vi "Power Qualtiy - 7 (Sub Vi).vi"(8 "Dynamic Data 6":dynamicdata(waveform)) -> (10 "Dynamic Data 2":dynamicdata(waveform), 12 "Dynamic Data":dynamicdata(waveform), 14 "Dynamic Data 4":dynamicdata(waveform), 15 "FFT - (RMS)":dynamicdata(waveform), 16 "Current":dbl(knob) scale=0.0..10.0, 17 "RMS":dynamicdata(waveform), 18 "Current Harmonics":dynamicdata(graph), 19 "IHD 7":dbl, 20 "Dynamic Data 3":dynamicdata(waveform), 21 "THD":dbl, 22 "Dynamic Data 5":dynamicdata(waveform), 23 "IHD 1":dbl, 24 "THD 2":dynamicdata(waveform), 25 "IHD 3":dbl, 26 "IHD 5":dbl)   [LabVIEW 2015]
uses:
  <vilib>/express/express analysis/Spectral/Block/exnSpectralBlock spectral measurements RMS poly.vi
  <vilib>/express/express analysis/Spectral/Block/exnSpectralBlock spectral measurements RMS DDT.vi
  <vilib>/express/express analysis/Spectral/XNode/ExpressSpectralMeasurementsBlockNode.xnode
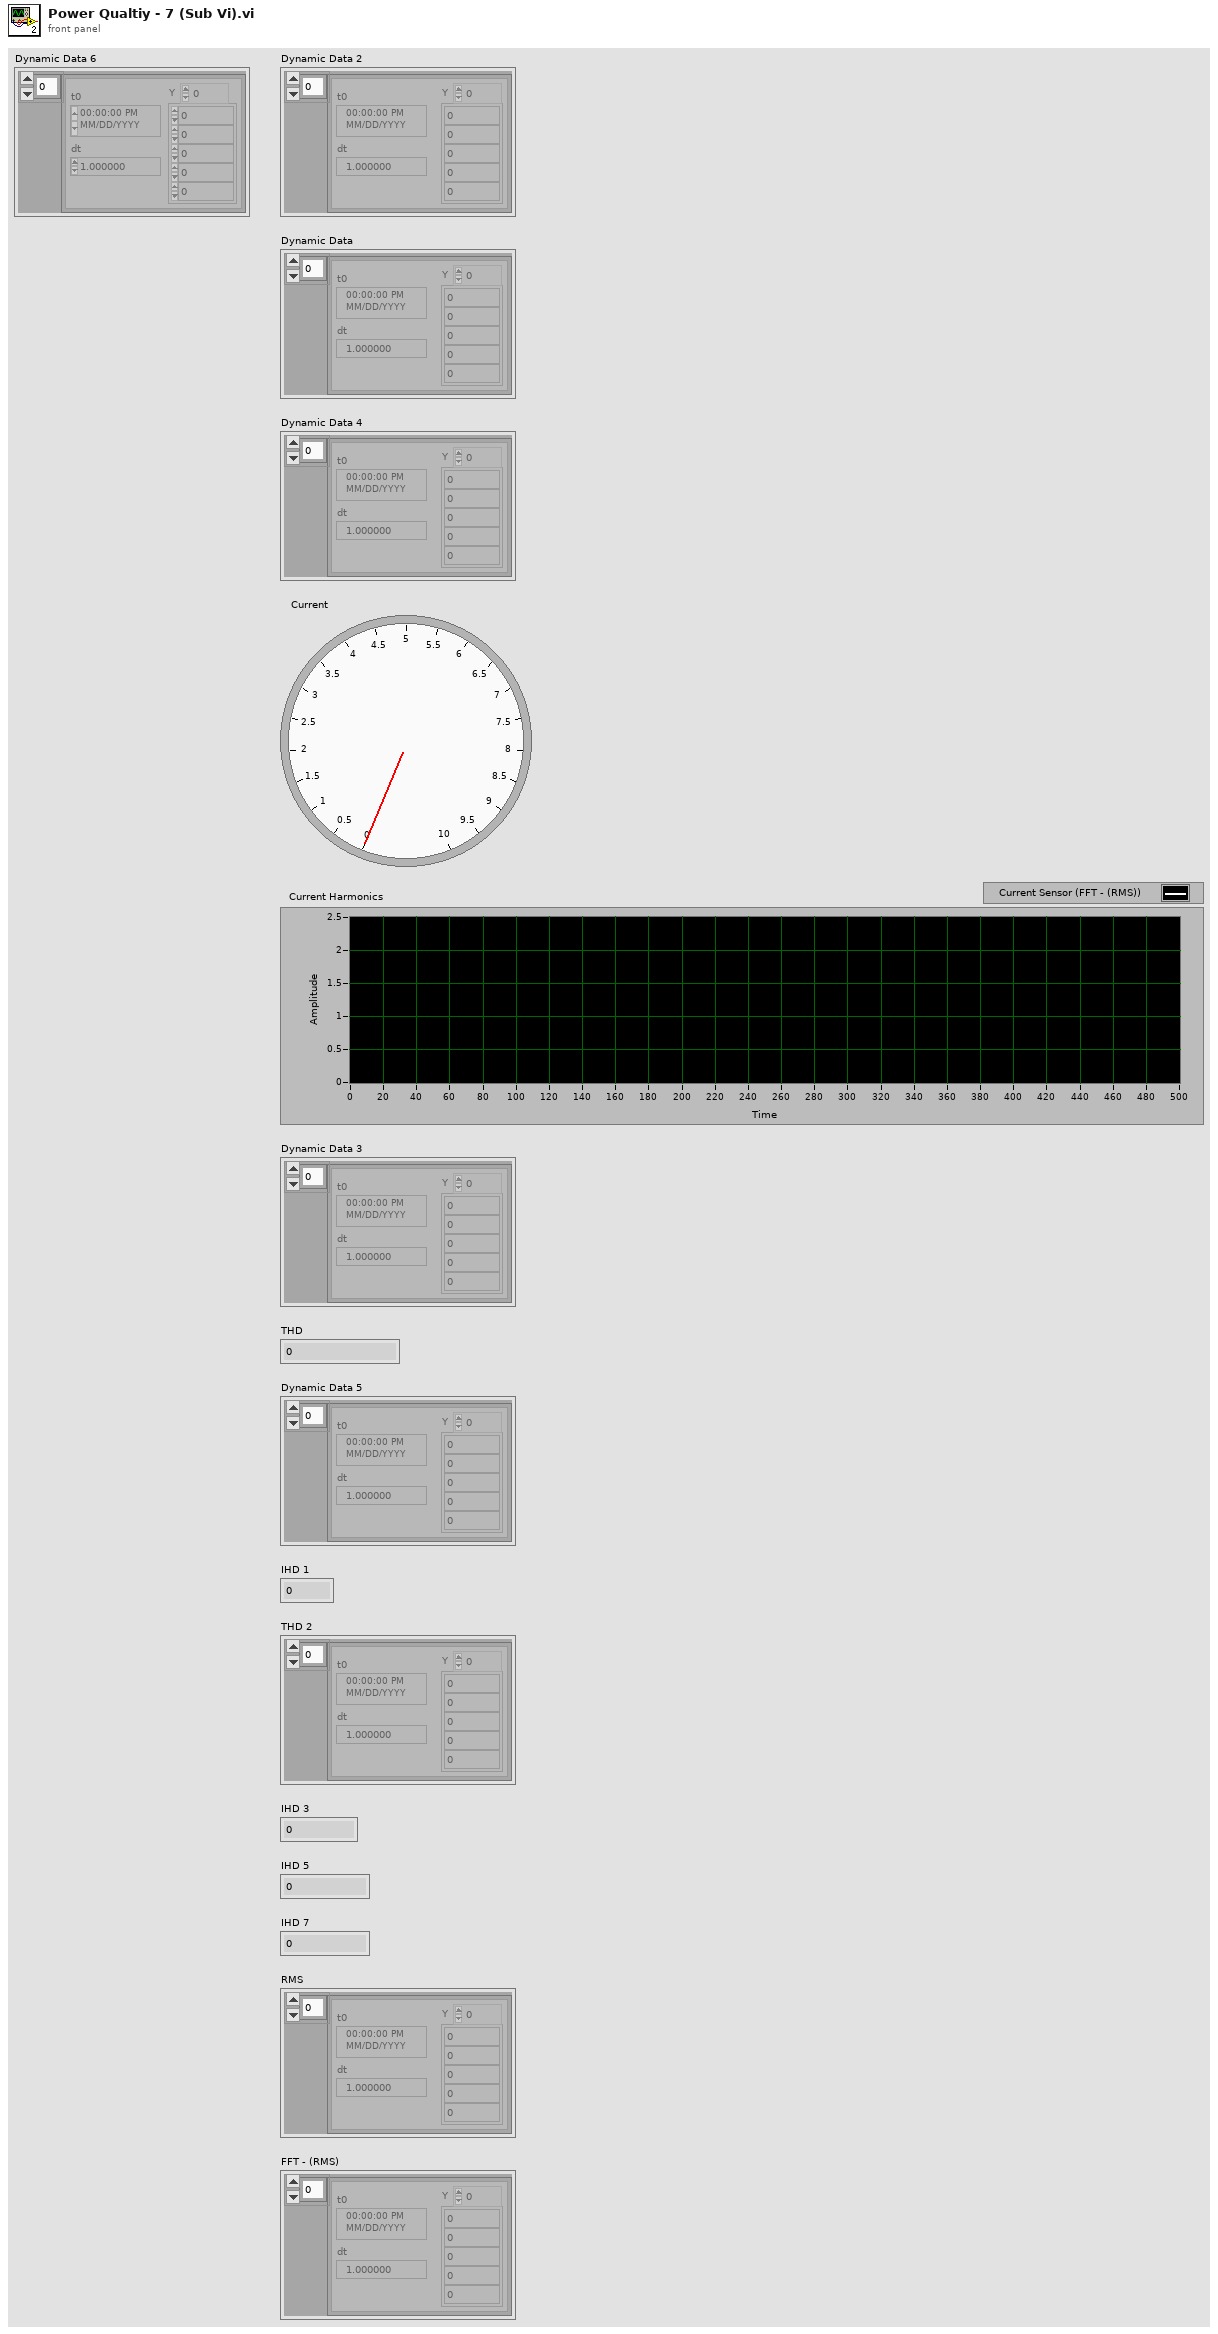
[diagram p1: front panel]
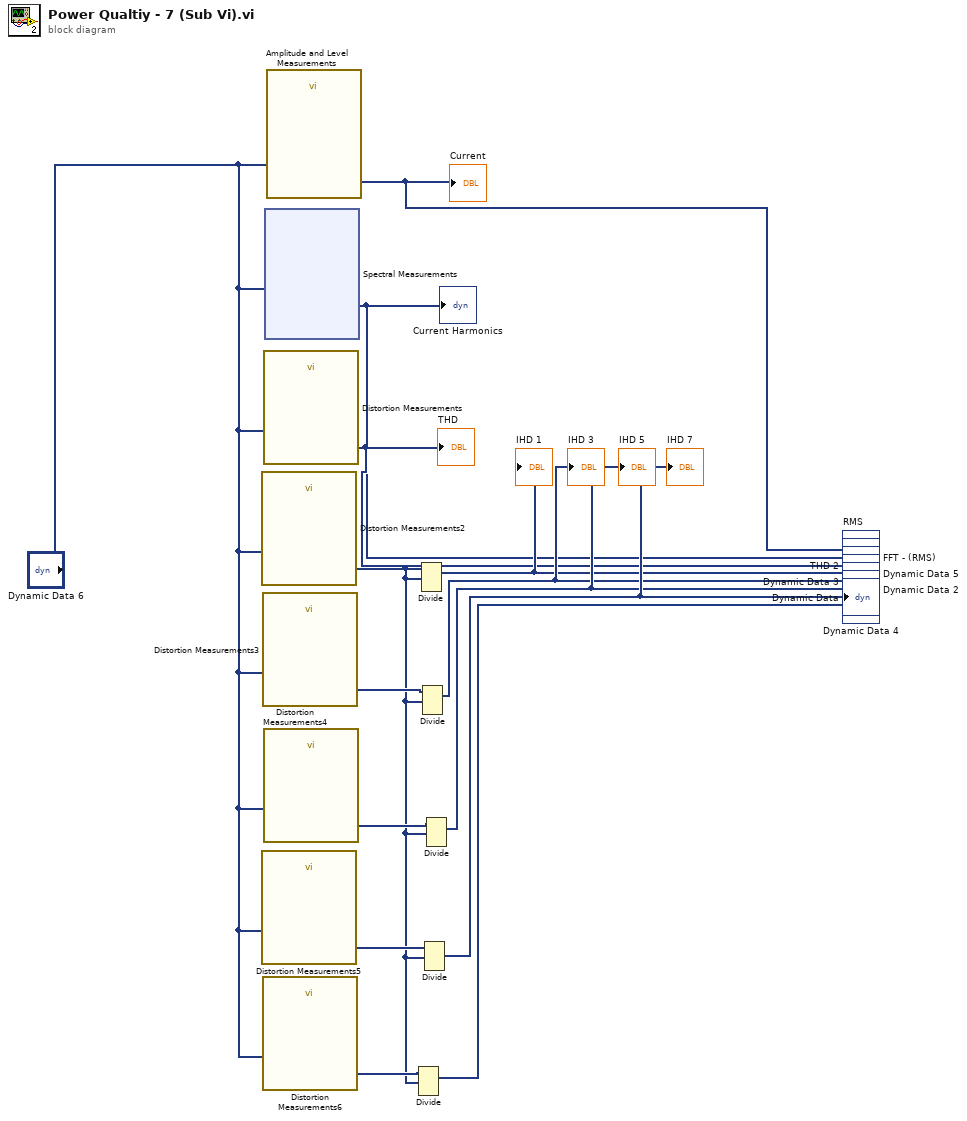
[diagram p0: block diagram]
diagram:
  n1 = call "Distortion Measurements2"("Signals"="Dynamic Data 6") -> ("Specific Harmonic"=w1:dynamicdata)  [unwired: 9 in, 1 out]
  n2 = call "Distortion Measurements5"("Signals"="Dynamic Data 6") -> ("Specific Harmonic"=w3:dynamicdata)  [unwired: 9 in, 1 out]
  n3 = call "Distortion Measurements3"("Signals"="Dynamic Data 6") -> ("Specific Harmonic"=w5:dynamicdata)  [unwired: 9 in, 1 out]
  n4 = call "Distortion Measurements6"("Signals"="Dynamic Data 6") -> ("Specific Harmonic"=w2:dynamicdata)  [unwired: 9 in, 1 out]
  n5 = call "Distortion Measurements"("Signals"="Dynamic Data 6") -> ("THD"=→"THD" →"THD 2":dynamicdata)  [unwired: 9 in, 1 out]
  n6 = call "Distortion Measurements4"("Signals"="Dynamic Data 6") -> ("Specific Harmonic"=w4:dynamicdata)  [unwired: 9 in, 1 out]
  n7 = xnode "Spectral Measurements"("Signals"="Dynamic Data 6") -> ("FFT - (RMS)"=→"Current Harmonics" →"FFT - (RMS)":dynamicdata)  [unwired: 1 in, 2 out]
  n8 = call "Amplitude and Level Measurements"("Signals"="Dynamic Data 6") -> ("RMS"=→"Current" →"RMS":dynamicdata)  [unwired: 13 in, 1 out]
  n9 = Divide(1:w1, 2:w2) -> (0:→"Dynamic Data 4":dynamicdata)  [unwired: 1 in, 1 out]
  n10 = Divide(1:w1, 2:w1) -> (0:→"IHD 1" →"Dynamic Data 5":dynamicdata)  [unwired: 1 in, 1 out]
  n11 = Divide(1:w1, 2:w5) -> (0:→"IHD 3" →"Dynamic Data 3":dynamicdata)  [unwired: 1 in, 1 out]
  n12 = Divide(1:w1, 2:w3) -> (0:→"IHD 7" →"Dynamic Data":dynamicdata)  [unwired: 1 in, 1 out]
  n13 = Divide(1:w1, 2:w4) -> (0:→"IHD 5" →"Dynamic Data 2":dynamicdata)  [unwired: 1 in, 1 out]
